vi "Write_Feedback_MsgQ.vi"(8 "error in (no error)":errorcluster, 9 "Code":dbl, 10 "Data in":string[](array[string])=[""], 11 "ResponseAddr":string="notif1") -> (0 "error out":errorcluster)   [LabVIEW 2019, in "MsgQ.lvlib"]
uses:
  MsgQ.lvlib
  mmw_Service/TypeDef/NotifierQ.ctl
  mmw_Service/Service.lvlib
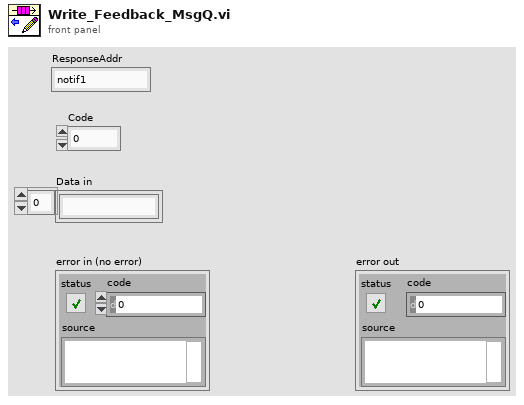
[diagram p1: front panel]
types:
  T1 = typedef "Service.lvlib/NotifierQ.ctl" = cluster{"Data":variant, "Code":dbl}
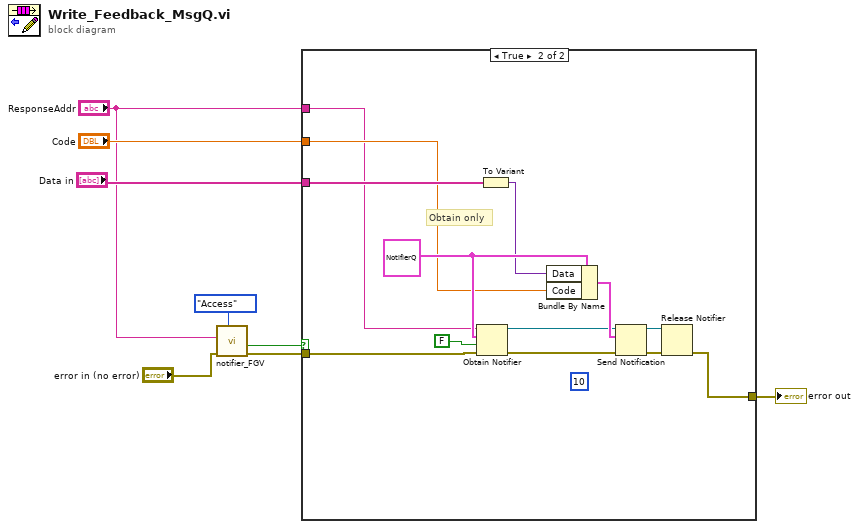
[diagram p0: block diagram]
diagram:
  n1 = call "notifier_FGV.vi"("Mode"=enum16{"Status", "Add", "Access", "Delete"}."Access", "error in (no error)"="error in (no error)", "ResponseAddr in"="ResponseAddr") -> ("error out"=w4:errorcluster, "Success?"=w1:bool)  [unwired: 5 in, 2 out]
  n2 = case shown="True" w1 {
    tunnel: [w9 w21] -> w8
    tunnel: "Data in" -> [_ w20]
    tunnel: "Code" -> [_ w13]
    tunnel: w4 -> [w9 w11]
    tunnel: "ResponseAddr" -> [_ w10]
    frame False {
    }
    frame True {
      w14 = T1 {"Data"=variant(enum16{""} enum.""), "Code"=0.0}
      (unwired) 10 ("timeout in ms (-1)")
      # "Obtain only"
      n3 = Obtain Notifier(name (unnamed)=w10, notification data type=w14, create if not found? (T)=FALSE, error in (no error)=w11) -> (notifier out=w15:refnum<notifier>, error out=w17:errorcluster)  [unwired: 1 out]
      n4 = To Variant(anything=w20) -> (Variant=w12:variant)
      n5 = Bundle By Name(cluster=w14, "Data"=w12, "Code"=w13) -> (w19:T1)
      n6 = Send Notification(notification=w19, notifier=w15, error in (no error)=w17) -> (notifier out=w18:refnum<notifier>, error out=w16:errorcluster)
      n7 = Release Notifier(notifier=w18, error in (no error)=w16) -> (error out=w21:errorcluster)  [unwired: 1 in, 2 out]
    }
  }
  "error out" <- w8
